vi "Create My API.vi"(5 "My API in":refnum<class "My API.lvclass">, 8 "error in (no error)":errorcluster, 11 "http-client (default)":refnum<class "httpClient.lvclass">) -> (0 "error out":errorcluster, 3 "My API out":refnum<class "My API.lvclass">)   [LabVIEW 2020, in "My API.lvclass"]
uses:
  My API.lvclass
  http-client-pkg/httpClient/httpClient.lvclass
  My API.lvclass/My API.ctl
  classes/REST Client/REST Client.lvclass
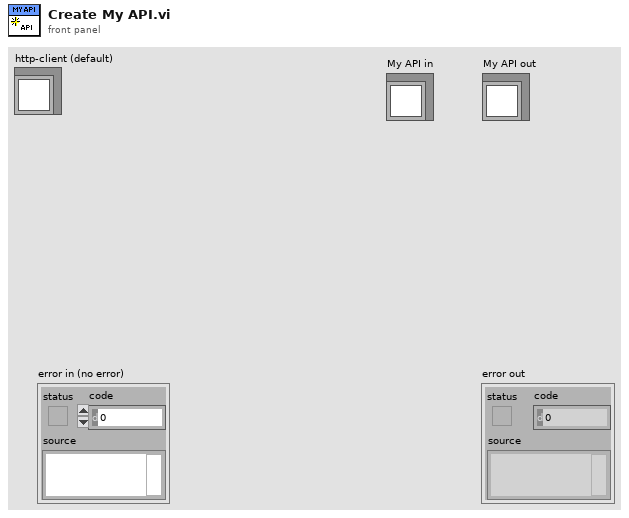
[diagram p1: front panel]
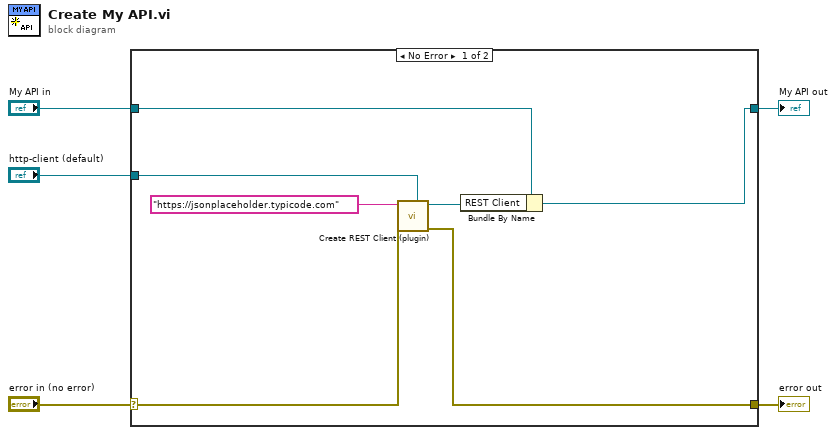
[diagram p0: block diagram]
diagram:
  n1 = case shown="No Error" "error in (no error)" {
    selector: "error in (no error)" -> [w7 w14]
    tunnel: [w8 w14] -> w4
    tunnel: [w9 w13] -> w2
    tunnel: "My API in" -> [w10 w13]
    tunnel: "http-client (default)" -> [w6 _]
    frame No Error {
      n2 = call "Create REST Client (plugin).vi"("http-client (default)"=w6, "error in (no error)"=w7, "Base URL"="https://jsonplaceholder.typicode.com") -> ("error out"=w8:errorcluster, "REST Client out"=w11:refnum<class "REST Client.lvclass">)  [unwired: 7 in]
      n3 = Bundle By Name(cluster=w10, "REST Client"=w11) -> (w9:refnum<class "My API.lvclass">)
    }
    frame Error {
    }
  }
  "error out" <- w4
  "My API out" <- w2
